vi "Teleop.vi"(10 "Match Info":T1={"Autonomous Elapsed Seconds"=0.0, "TeleOp Elapsed Seconds"=118.321, "Disabled Elapsed Seconds"=65.439, "Visited Autonomous"=FALSE, "Visited TeleOp"=TRUE, "Visited Disabled"=TRUE, "Autonomous Settings"={"Autonomous Style"=enum."Independent", "VI Refnum"=refnum}}, 11 "Call Context":T2=enum."Execute") -> ()   [LabVIEW 2015]
doc: "This VI is called for each TeleOp packet received from the DS where the robot is not disabled. It is often used to read from the joysticks and update I/O or to update setpoints for timed control loops. It should complete and return within 20 milliseconds or it may miss DS packets."
uses:
  <vilib>/Rock Robotics/WPI/DriverStation/WPI_DriverStationDerivedRobotMode.ctl
  <vilib>/Rock Robotics/WPI/DriverStation/WPI_DriverStationMatch Info.ctl
  <vilib>/Rock Robotics/WPI/Solenoid/WPI_SolenoidValue.ctl
  <vilib>/Rock Robotics/WPI/Utilities/WPI_GetSetVariantRefNum.vi
  <vilib>/Rock Robotics/WPI/Solenoid/WPI_SolenoidSetEnum.vi
panel:
  in  "Forza style":bool=TRUE
  in  "Toggle cheval":i32=2 min=0 max=9 step=1
  in  "Toggle Lanceur":i32=3 min=0 max=9 step=1
  in  "Take button":i32=5 min=0 max=9 step=1
  in  "Shoot button":i32=4 min=0 max=9 step=1
  in  "Stop button":i32=1 min=0 max=9 step=1
  in  "Take Speed":dbl=0.39999999999999997 min=0.0 max=1.0 step=0.05 format="%#_13g"
  in  "Shoot Speed":dbl=0.9 min=0.0 max=1.0 step=0.05
  # "Lanceur"
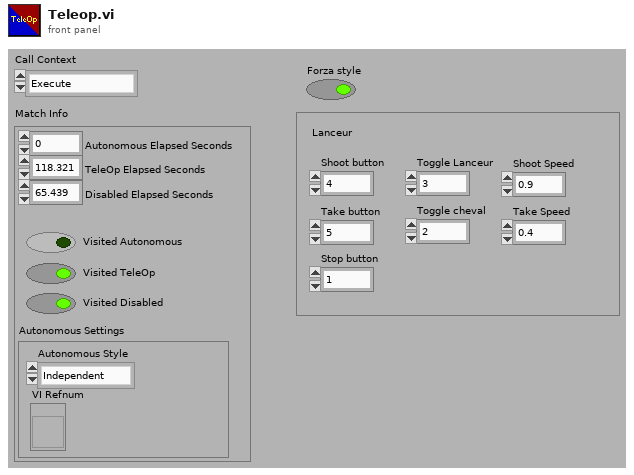
[diagram p1: front panel]
types:
  T1 = typedef "WPI_DriverStationMatch Info.ctl" = cluster{"Autonomous Elapsed Seconds":dbl, "TeleOp Elapsed Seconds":dbl, "Disabled Elapsed Seconds":dbl, "Visited Autonomous":bool, "Visited TeleOp":bool, "Visited Disabled":bool, "Autonomous Settings":cluster{"Autonomous Style":enum16{"Iterative", "Independent"}, "VI Refnum":refnum<vi>}}
  T2 = typedef "WPI_DriverStationDerivedRobotMode.ctl" = enum16{"Init", "Execute", "Stop"}
  T3 = typedef "WPI_SolenoidValue.ctl" = enum16{"Off", "On", "Forward", "Reverse"}
  T4 = typedef "WPI_JoystickDevRef.ctl" = cluster{"Device":T5}
  T5 = typedef "WPI_JoystickDeviceEnum.ctl" = enum16{"USB 0", "USB 1", "USB 2", "USB 3", "USB 4", "USB 5"}
  T6 = cluster{"Axes[0]":dbl, "Axes[1]":dbl, "Axes[2]":dbl, "Axes[3]":dbl, "Axes[4]":dbl, "Axes[5]":dbl, "Axes[6]":dbl, "Axes[7]":dbl, "Axes[8]":dbl}
  T7 = typedef "WPI_MotorControlDeviceRef.ctl" = cluster{"DeviceStatus":errorcluster, "Type":T8, "PWM":cluster{"PWM Channel":T9, "DeadBand":T10}, "CAN":cluster{"Device Number":u8, "Control Mode":T11, "Semaphore":T12, "Max Vout":dbl, "TalonSRX Control Mode":T13}, "Invert":bool}
  T8 = typedef "WPI_MotorControlType.ctl" = enum16{"PWM", "CAN", "CANTalonSRX"}
  T9 = typedef "FPGA_DIOPWMChannel.ctl" = enum8{"PWM 0", "PWM 1", "PWM 2", "PWM 3", "PWM 4", "PWM 5", "PWM 6", "PWM 7", "PWM 8", "PWM 9", "PWM MXP 0", "PWM MXP 1", "PWM MXP 2", "PWM MXP 3", "PWM MXP 4", "PWM MXP 5", "PWM MXP 6", "PWM MXP 7", "PWM MXP 8", "PWM MXP 9", "Invalid"}
  T10 = typedef "WPI_PWMDeadband.ctl" = cluster{"Name":string, "maxPositivePwm":i32, "minPositivePwm":i32, "centerPwm":i32, "maxNegativePwm":i32, "minNegativePwm":i32, "angularRange":u16}
  T11 = typedef "WPI_CANJaguar_ControlMode.ctl" = enum8{"Percent VBus", "Current", "Speed", "Position", "Voltage"}
  T12 = typedef "Semaphore RefNum" = refnum<k1>
  T13 = typedef "WPI_CANTalonSRX_APIControlMode.ctl" = enum8{"Percent VBus", "Speed", "Position", "Slave", "Unchanged / Invalid", "Voltage Compensation", "Current", "Motion Profile"}
  T14 = typedef "WPI_RobotDriveDevRef.ctl" = cluster{"DevStatus":errorcluster, "Motors[]":T7[], "Square Inputs":bool, "Max Output":dbl}
  T15 = typedef "WPI_SolenoidDevRef.ctl" = cluster{"DevStatus":errorcluster, "Pneumatics Control Module":u8, "Forward Solenoid Channel":T16, "Reverse Solenoid Channel":T16}
  T16 = typedef "WPI_SolenoidChannel.ctl" = enum8{"Solenoid 0", "Solenoid 1", "Solenoid 2", "Solenoid 3", "Solenoid 4", "Solenoid 5", "Solenoid 6", "Solenoid 7", "Invalid"}
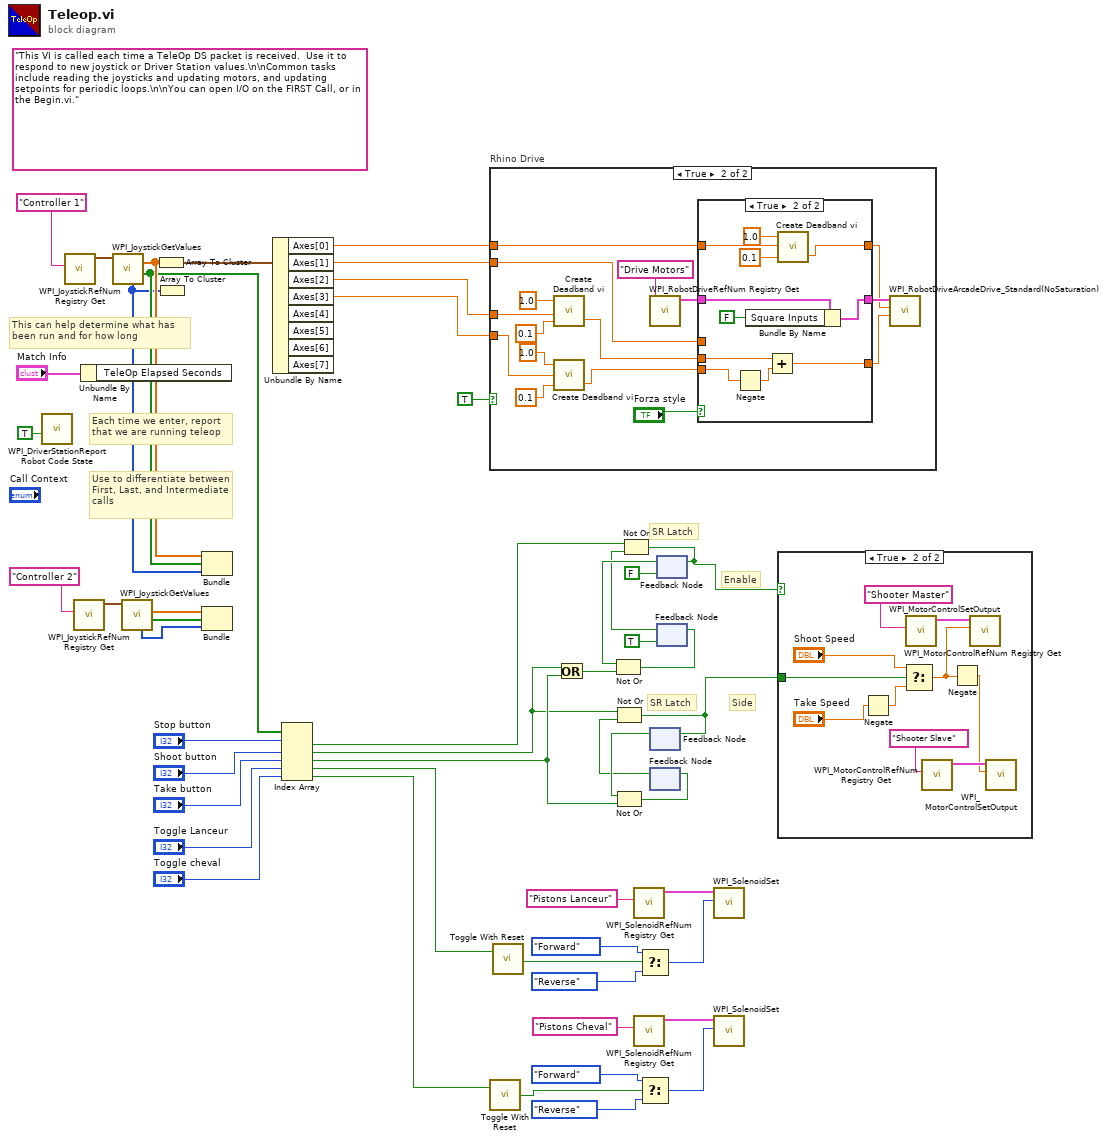
[diagram p0: block diagram]
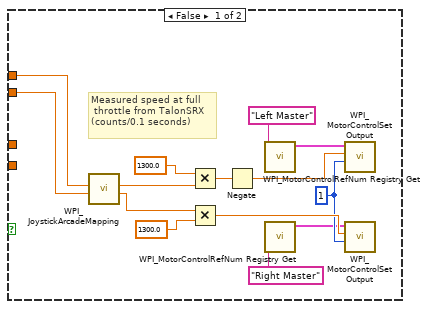
[diagram p2: hidden frame]
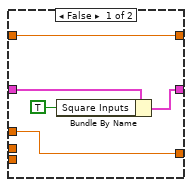
[diagram p3: hidden frame]
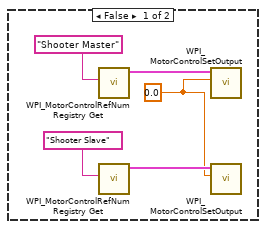
[diagram p4: hidden frame]
diagram:
  (unwired) "This VI is called each time a TeleOp DS packet is received.  Use it to respond to new joystick or Driver Station values.\n\nCommon tasks include reading the joysticks and updating motors, and updating setpoints for periodic loops.\n\nYou can open I/O on the FIRST Call, or in the Begin.vi."
  # "Side"
  # "Enable"
  # "SR Latch"
  # "SR Latch"
  # "Each time we enter, report that we are running teleop"
  # "Use to differentiate between First, Last, and Intermediate calls"
  # "This can help determine what has\nbeen run and for how long"
  n1 = call <vilib>:"WPI_DriverStationReport Robot Code State.vi"("TeleOp"=TRUE ("Autonomous")) -> ()  [unwired: 10 in, 1 out]
  n2 = call <vilib>:"WPI_JoystickRefNum Registry Get.vi"("refnum name"="Controller 1") -> ("JoystickDevRef"=w49:T4)  [unwired: 1 in, 9 out]
  n3 = call <vilib>:"WPI_JoystickRefNum Registry Get.vi"("refnum name"="Controller 2") -> ("JoystickDevRef"=w6:T4)  [unwired: 1 in, 9 out]
  n4 = Unbundle By Name("Match Info") -> ()  [unwired: 1 out]
  n5 = call <vilib>:"WPI_JoystickGetValues.vi"("JoystickDevRef"=w49) -> ("Buttons"=w8:bool[], "Axes"=w9:dbl[], "POVs"=w7:i16[])  [unwired: 6 in, 2 out]
  n6 = call <vilib>:"WPI_JoystickGetValues.vi"("JoystickDevRef"=w6) -> ("Buttons"=w3:bool[], "Axes"=w4:dbl[], "POVs"=w2:i16[])  [unwired: 6 in, 2 out]
  n7 = Array To Cluster(array=w9) -> (cluster=w47:T6)
  n8 = Array To Cluster(array=w7) -> ()  [unwired: 1 out]
  n9 = Bundle("Axes"=w9, "Buttons"=w8, "POVs"=w7) -> ()  [unwired: 1 in, 1 out]
  n10 = Bundle("Axes"=w4, "Buttons"=w3, "POVs"=w2) -> ()  [unwired: 1 in, 1 out]
  n11 = Unbundle By Name(w47) -> ("Axes[0]"=w27:dbl, "Axes[1]"=w28:dbl, "Axes[2]"=w24:dbl, "Axes[3]"=w23:dbl)  [unwired: 4 out]
  n12 = Index Array(array=w8, index #1="Stop button", index #2="Shoot button", index #3="Take button", index #4="Toggle Lanceur", index #5="Toggle cheval") -> (element #1=w29:bool, element #2=w32:bool, element #3=w33:bool, element #4=w22:bool, element #5=w21:bool)
  n13 = case "Rhino Drive" shown="True" TRUE {
    tunnel: w28 -> [w52 w79]
    tunnel: w27 -> [w53 w67]
    tunnel: w24 -> [_ w71]
    tunnel: w23 -> [_ w75]
    frame False {
      w60 = u8 1 ("Sync Group / Parameter Slot")
      # "Measured speed at full\n throttle from TalonSRX\n(counts/0.1 seconds)"
      n14 = call <vilib>:"WPI_JoystickArcadeMapping.vi"("Y axis value"=w52, "X axis value"=w53) -> ("Right Motor Value"=w55:dbl, "Left Motor Value"=w54:dbl)  [unwired: 8 in]
      n15 = Multiply(x=1300.0, y=w54) -> (x*y=w61:dbl)
      n16 = Multiply(x=w55, y=1300.0) -> (x*y=w63:dbl)
      n17 = Negate(x=w61) -> (-x=w62:dbl)
      n18 = call <vilib>:"WPI_MotorControlRefNum Registry Get.vi"("refnum name"="Left Master") -> ("MotorControlDevRef"=w58:T7)  [unwired: 9 in, 1 out]
      n19 = call <vilib>:"WPI_MotorControlRefNum Registry Get.vi"("refnum name"="Right Master") -> ("MotorControlDevRef"=w59:T7)  [unwired: 9 in, 1 out]
      n20 = call <vilib>:"WPI_MotorControlSetOutput.vi"("Sync Group / Parameter Slot"=w60, "Output"=w62, "MotorControlDevRef"=w58) -> ()  [unwired: 6 in, 3 out]
      n21 = call <vilib>:"WPI_MotorControlSetOutput.vi"("Sync Group / Parameter Slot"=w60, "Output"=w63, "MotorControlDevRef"=w59) -> ()  [unwired: 6 in, 3 out]
    }
    frame True {
      n22 = call "Create Deadband vi.vi"("Input Deadband"=0.1, "Input"=w71, "Output Upper Limit"=1.0) -> ("Output"=w70:dbl)  [unwired: 1 in]
      n23 = call "Create Deadband vi.vi"("Input Deadband"=0.1, "Input"=w75, "Output Upper Limit"=1.0) -> ("Output"=w74:dbl)  [unwired: 1 in]
      n24 = call <vilib>:"WPI_RobotDriveRefNum Registry Get.vi"("refnum name"="Drive Motors") -> ("RobotDriveDevRef"=w77:T14)  [unwired: 1 in, 9 out]
      n25 = case shown="True" "Forza style" {
        tunnel: w70 -> [_ w95]
        tunnel: w74 -> [_ w96]
        tunnel: [w86 w94] -> w80
        tunnel: w79 -> [w86 _]
        tunnel: w77 -> [w84 w93]
        tunnel: [w85 w92] -> w76
        tunnel: w67 -> [w82 w90]
        tunnel: [w82 w89] -> w66
        frame False {
          n26 = Bundle By Name(cluster=w84, "Square Inputs"=TRUE) -> (w85:T14)
        }
        frame True {
          n27 = Negate(x=w96) -> (-x=w97:dbl)
          n28 = Bundle By Name(cluster=w93, "Square Inputs"=FALSE) -> (w92:T14)
          n29 = Add(x=w95, y=w97) -> (x+y=w94:dbl)
          n30 = call "Create Deadband vi.vi"("Input Deadband"=0.1, "Input"=w90, "Output Upper Limit"=1.0) -> ("Output"=w89:dbl)  [unwired: 1 in]
        }
      }
      n31 = call <vilib>:"WPI_RobotDriveArcadeDrive_Standard(NoSaturation).vi"("Y axis value"=w80, "X axis value"=w66, "RobotDriveDevRef"=w76) -> ()  [unwired: 1 in, 8 out]
    }
  }
  n32 = call "Toggle With Reset.vi"("Boolean"=w21) -> ("Driver Switch 2"=w1:bool)  [unwired: 1 in]
  n33 = call "Toggle With Reset.vi"("Boolean"=w22) -> ("Driver Switch 2"=w10:bool)  [unwired: 1 in]
  n34 = Or(x=w32, y=w33) -> (x .or. y?=w39:bool)
  n35 = call <vilib>:"WPI_SolenoidRefNum Registry Get.vi"("refnum name"="Pistons Lanceur") -> ("SolenoidDevRef"=w18:T15)  [unwired: 9 in, 1 out]
  n36 = call <vilib>:"WPI_SolenoidRefNum Registry Get.vi"("refnum name"="Pistons Cheval") -> ("SolenoidDevRef"=w14:T15)  [unwired: 9 in, 1 out]
  n37 = Select(t=WPI_SolenoidValue."Forward" ("Value"), s=w10, f=WPI_SolenoidValue."Reverse" ("Value")) -> (s? t:f=w20:T3)
  n38 = Select(t=WPI_SolenoidValue."Forward" ("Value"), s=w1, f=WPI_SolenoidValue."Reverse" ("Value")) -> (s? t:f=w12:T3)
  n39 = feedback #1() -> (w46:bool)  [unwired: 1 in]
  n40 = Not Or(1:w33, 2:w46) -> (0:w45:bool)
  n41 = feedback #2() -> (w44:bool)  [unwired: 1 in]
  n42 = Not Or(1:w44, 2:w32) -> (0:w43:bool)
  n43 = feedback-in #1(w43) -> ()
  n44 = feedback-in #2(w45) -> ()
  n45 = feedback #3(FALSE) -> (w42:bool)
  n46 = Not Or(1:w39, 2:w42) -> (0:w41:bool)
  n47 = feedback #4(TRUE) -> (w40:bool)
  n48 = Not Or(1:w40, 2:w29) -> (0:w25:bool)
  n49 = feedback-in #3(w25) -> ()
  n50 = feedback-in #4(w41) -> ()
  n51 = call-poly <vilib>:"WPI_SolenoidSet.vi"("Value"=w20, "SolenoidDevRef"=w18) -> ()  [unwired: 8 in, 2 out]
  n52 = call-poly <vilib>:"WPI_SolenoidSet.vi"("Value"=w12, "SolenoidDevRef"=w14) -> ()  [unwired: 8 in, 2 out]
  n53 = case shown="True" w25 {
    tunnel: w43 -> [_ w110]
    frame False {
      w98 = 0.0 ("Output")
      n54 = call <vilib>:"WPI_MotorControlRefNum Registry Get.vi"("refnum name"="Shooter Master") -> ("MotorControlDevRef"=w102:T7)  [unwired: 9 in, 1 out]
      n55 = call <vilib>:"WPI_MotorControlRefNum Registry Get.vi"("refnum name"="Shooter Slave") -> ("MotorControlDevRef"=w99:T7)  [unwired: 9 in, 1 out]
      n56 = call <vilib>:"WPI_MotorControlSetOutput.vi"("Output"=w98, "MotorControlDevRef"=w102) -> ()  [unwired: 7 in, 3 out]
      n57 = call <vilib>:"WPI_MotorControlSetOutput.vi"("Output"=w98, "MotorControlDevRef"=w99) -> ()  [unwired: 7 in, 3 out]
    }
    frame True {
      n58 = Negate(x="Take Speed") -> (-x=w107:dbl)
      n59 = Select(t="Shoot Speed", s=w110, f=w107) -> (s? t:f=w105:dbl)
      n60 = call <vilib>:"WPI_MotorControlRefNum Registry Get.vi"("refnum name"="Shooter Master") -> ("MotorControlDevRef"=w111:T7)  [unwired: 9 in, 1 out]
      n61 = call <vilib>:"WPI_MotorControlRefNum Registry Get.vi"("refnum name"="Shooter Slave") -> ("MotorControlDevRef"=w106:T7)  [unwired: 9 in, 1 out]
      n62 = Negate(x=w105) -> (-x=w103:dbl)
      n63 = call <vilib>:"WPI_MotorControlSetOutput.vi"("Output"=w105, "MotorControlDevRef"=w111) -> ()  [unwired: 7 in, 3 out]
      n64 = call <vilib>:"WPI_MotorControlSetOutput.vi"("Output"=w103, "MotorControlDevRef"=w106) -> ()  [unwired: 7 in, 3 out]
    }
  }
